vi "Add Log File - Right Click.vi"() -> ()   [LabVIEW 2012, in "Waveform Data Logger System Explorer.lvlib"]
uses:
  Waveform Data Logger System Explorer.lvlib
  <vilib>/NI Veristand/Custom Device API/Custom Device Item Ref.ctl
  <vilib>/NI VeriStand/Custom Device API/Custom Device API.lvlib
panel:
  in  "Node Ptr":T1=18446744073709551615 format="%.0x"
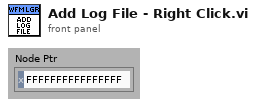
[diagram p1: front panel]
types:
  T1 = typedef "Custom Device API.lvlib/Custom Device Item Ref.ctl" = u64
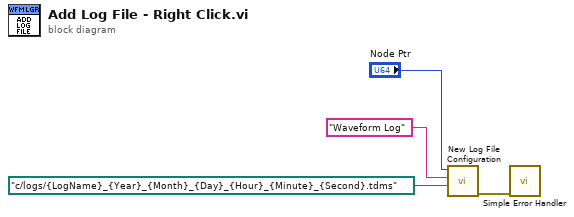
[diagram p0: block diagram]
diagram:
  n1 = call "New Log File Configuration.vi"("Default Path"=path "c:/logs/{LogName}_{Year}_{Month}_{Day}_{Hour}_{Minute}_{Second}.tdms" ("Default Log Directory"), "Default Name"="Waveform Log", "Device Ref in"="Node Ptr") -> ("error out"=w1:errorcluster)  [unwired: 1 in, 7 out]
  n2 = call <vilib>:"Simple Error Handler.vi"("error in (no error)"=w1) -> ()  [unwired: 4 in, 5 out]
